vi "Stellarnet_spectrometer_Full_acquire_spectra.vi"() -> ()   [LabVIEW 2014]
uses:
  <vilib>/Utility/file.llb/Write To Spreadsheet File (string).vi
  <vilib>/Utility/file.llb/Write To Spreadsheet File (DBL).vi
panel:
  out "output param":i32
  out "Critical Error":bool
  out "Spectrum":cluster{"Wavelengths":dbl[], "buffer out":sgl[]}(graph)
  in  "Save spectra file path":path=path "C:/Users/User/Desktop/Chamber Data/perovskites/2015-08-04 spectra"
  in  "spectra settings":i32[](array[numeric]) caption="Integration time (ms)\n\nOptical smoothing level\n\nNumber of scans to average\n\nDigitizer clock rate setting" min=0 max=4 step=1
  in  "Aquire spectra":bool
  in  "Seconds between  spectra":dbl caption="Time Target (s)"
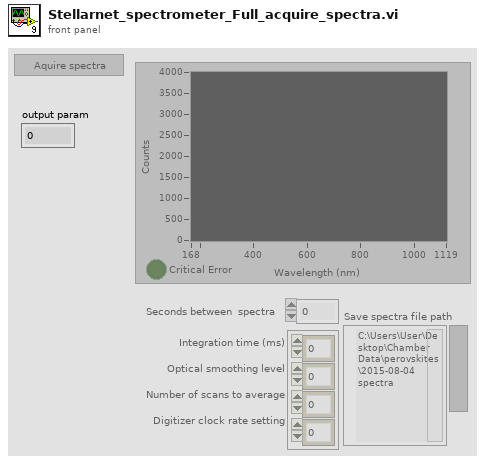
[diagram p1: front panel]
types:
  T1 = enum8{"Enabled", "Disabled", "Disabled and Grayed Out"}
  T2 = cluster{"Coefficients":ext[], "Wavelengths":dbl[]}[]
  T3 = cluster{"Integration Time (ms)":i32, "Number of Scans to Average":i32, "Optical Smoothing Level":i32, "Digitizer Clock Rate Setting":i32, "Temp  Compensation ":bool}[]
  T4 = cluster{"Integration Time (ms)":i32, "Number of Scans to Average":i32, "Optical Smoothing Level":i32, "Digitizer Clock Rate Setting":i32, "Temp  Compensation ":bool}
  T5 = cluster{"Coefficients":ext[], "Wavelengths":dbl[]}
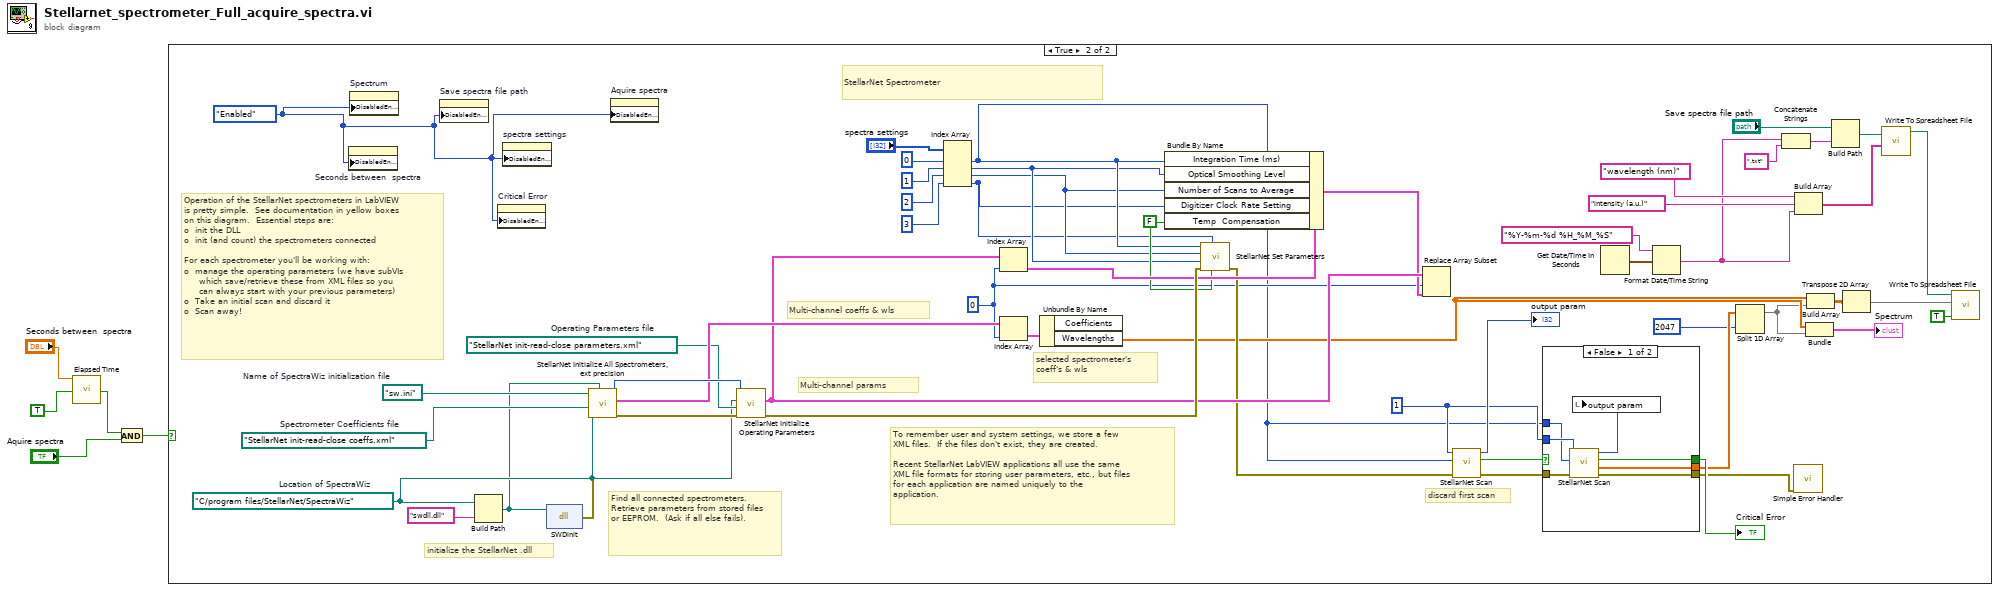
[diagram p0: block diagram]
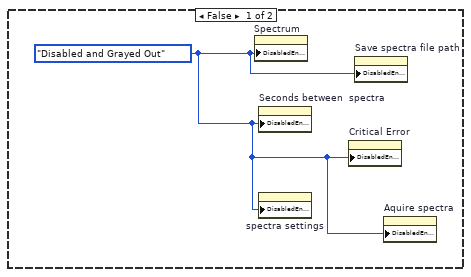
[diagram p2: hidden frame]
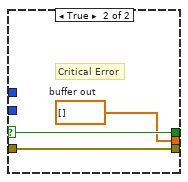
[diagram p3: hidden frame]
diagram:
  n1 = call "Elapsed Time"("Time Target (s)"="Seconds between  spectra", "Auto Reset"=TRUE) -> ("Time has Elapsed"=w3:bool)  [unwired: 10 in, 7 out]
  n2 = And(x=w3, y="Aquire spectra") -> (x .and. y?=w1:bool)
  n3 = case shown="True" w1 {
    frame False {
      w6 = T1."Disabled and Grayed Out" ("Disabled")
      n4 = property on="Spectrum" class="XYGraph (strict)"("DisabledEnum"=w6) -> ()  [unwired: 2 in, 2 out]
      n5 = property on="Seconds between  spectra" class="DigNum (strict)"("DisabledEnum"=w6) -> ()  [unwired: 2 in, 2 out]
      n6 = property on="spectra settings" class="Arr (strict)"("DisabledEnum"=w6) -> ()  [unwired: 2 in, 2 out]
      n7 = property on="Critical Error" class="Bool (strict)"("DisabledEnum"=w6) -> ()  [unwired: 2 in, 2 out]
      n8 = property on="Save spectra file path" class="Path"("DisabledEnum"=w6) -> ()  [unwired: 2 in, 2 out]
      n9 = property on="Aquire spectra" class="Bool (strict)"("DisabledEnum"=w6) -> ()  [unwired: 2 in, 2 out]
    }
    frame True {
      w7 = T1."Enabled" ("Disabled")
      w31 = 0 ("Spectral Channel")
      w33 = 1 ("Spectral Channel")
      w37 = FALSE ("Temp  Compensation")
      w41 = path "C:/program files/StellarNet/SpectraWiz"  # Location of SpectraWiz
      w51 = path "sw.ini"  # Name of SpectraWiz initialization file
      w43 = path "StellarNet init-read-close parameters.xml"  # Operating Parameters file
      w52 = path "StellarNet init-read-close coeffs.xml"  # Spectrometer Coefficients file
      # "StellarNet Spectrometer"
      # "Operation of the StellarNet spectrometers in LabVIEW\nis pretty simple.  See documentation in yellow boxes\non this diagram.  Essential steps are:\no  init the DLL\no  init (and count) the spectrometers connected\n\nFor each spectrometer you'll be working with:\no  manage the operating parameters (we have subVIs\n     which save/retrieve these from XML files so you\n     can always start with your previous parameters)\no  Take an initial scan and discard it\no  Scan away!"
      # "initialize the StellarNet .dll"
      # "To remember user and system settings, we store a few \nXML files.  If the files don't exist, they are created.\n\nRecent StellarNet LabVIEW applications all use the same\nXML file formats for storing user parameters, etc., but files\nfor each application are named uniquely to the \napplication."
      # "Find all connected spectrometers.  Retrieve parameters from stored files or EEPROM.  (Ask if all else fails)."
      # "selected spectrometer's\ncoeff's & wls"
      # "Multi-channel coeffs & wls"
      # "Multi-channel params"
      # "discard first scan"
      n10 = property on="Seconds between  spectra" class="DigNum (strict)"("DisabledEnum"=w7) -> ()  [unwired: 2 in, 2 out]
      n11 = property on="Spectrum" class="XYGraph (strict)"("DisabledEnum"=w7) -> ()  [unwired: 2 in, 2 out]
      n12 = property on="Save spectra file path" class="Path"("DisabledEnum"=w7) -> ()  [unwired: 2 in, 2 out]
      n13 = Build Path(base path=w41, name or relative path="swdll.dll") -> (appended path=w39:path)
      n14 = property on="Critical Error" class="Bool (strict)"("DisabledEnum"=w7) -> ()  [unwired: 2 in, 2 out]
      n15 = property on="spectra settings" class="Arr (strict)"("DisabledEnum"=w7) -> ()  [unwired: 2 in, 2 out]
      n16 = dll-call lib="C:/Program Files/StellarNet/SpectraWiz/swdll.dll" fn="SWDinit" label="init"(path in=w39) -> (error out=w40:errorcluster)  [unwired: 3 in, 1 out]
      n17 = call "StellarNet Initialize All Spectrometers, ext precision.vi"("Path of swdll.dll"=w39, "error in"=w40, "Spectrometer Coefficients file"=w52, "Location of SpectraWiz"=w41, "Name of SpectraWiz initialization file"=w51) -> ("error out"=w50:errorcluster, "Multi Channel Coeffs & WLs"=w48:T2, "Number of Channels"=w49:i32)  [unwired: 2 in, 2 out]
      n18 = property on="Aquire spectra" class="Bool (strict)"("DisabledEnum"=w7) -> ()  [unwired: 2 in, 2 out]
      n19 = call "StellarNet Initialize Operating Parameters.vi"("error in"=w50, "Spectrometer Coefficients file"=w43, "Location of SpectraWiz"=w41, "Number of Channels"=w49) -> ("error out"=w46:errorcluster, "Operating Parameters"=w44:T3)  [unwired: 6 in]
      n20 = Index Array(array="spectra settings", index #1=0 ("index"), index #2=1 ("index"), index #3=2 ("index"), index #4=3 ("index")) -> (element #1=w11:i32, element #2=w10:i32, element #3=w9:i32, element #4=w8:i32)
      n21 = Index Array(array=w44, index=w31) -> (element=w45:T4)
      n22 = Index Array(array=w48, index=w31) -> (element=w47:T5)
      n23 = Unbundle By Name(w47) -> ("Wavelengths"=w35:dbl[])  [unwired: 1 out]
      n24 = Bundle By Name(cluster=w45, "Integration Time (ms)"=w11, "Optical Smoothing Level"=w10, "Number of Scans to Average"=w9, "Digitizer Clock Rate Setting"=w8, "Temp  Compensation"=w37) -> (w38:T4)
      n25 = call "StellarNet Set Parameters.vi"("Temp  Compensation"=w37, "Digitizer Clock Rate Setting"=w8, "error in (no error)"=w46, "Optical Smoothing Level"=w10, "Number of Scans to Average"=w9, "Integration Time (ms)"=w11) -> ("error out"=w36:errorcluster)  [unwired: 5 in]
      n26 = Replace Array Subset(array=w44, new element=w38, index=w31) -> ()  [unwired: 1 out]
      n27 = call "StellarNet Scan.vi"("error in (no error)"=w36, "Integration Time (msec)"=w11, "Spectral Channel"=w33) -> ("error out"=w57:errorcluster, "Critical Error"=w58:bool, "output param"=→"output param":i32)  [unwired: 5 in, 1 out]
      n28 = case shown="False" w58 {
        selector: w58 -> [_ w69]
        tunnel: w33 -> [w66 _]
        tunnel: [w65 w68] -> w42
        tunnel: [w63 w69] -> w55
        tunnel: w57 -> [w62 w67]
        tunnel: [w61 w67] -> w32
        tunnel: w11 -> [w60 _]
        frame False {
          n29 = call "StellarNet Scan.vi"("error in (no error)"=w62, "Integration Time (msec)"=w60, "Spectral Channel"=w66) -> ("error out"=w61:errorcluster, "buffer out"=w65:sgl[], "Critical Error"=w63:bool, "output param"=w64:i32)  [unwired: 5 in]
          n30 = local write "output param"(w64) -> ()
        }
        frame True {
          w68 = sgl[] []  # buffer out
          # "Critical Error"
        }
      }
      "Critical Error" <- w55
      n31 = Get Date/Time In Seconds() -> (seconds since 1Jan1904=w26:timestamp)
      n32 = Format Date/Time String(time format string (%c)="%Y-%m-%d %H_%M_%S", seconds (now)=w26) -> (date/time string=w21:string)  [unwired: 1 in]
      n33 = Split 1D Array(array=w42, index=2047) -> (first subarray=w34:sgl[])  [unwired: 1 out]
      n34 = Concatenate Strings(w21, ".txt") -> (w22:string)
      n35 = call <vilib>:"Simple Error Handler.vi"("error in (no error)"=w32) -> ()  [unwired: 4 in, 5 out]
      n36 = Build Array("wavelength (nm)", "intensity (a.u.)", w21) -> (w17:string[])
      n37 = Bundle("Wavelengths"=w35, w34) -> (→"Spectrum":cluster{"Wavelengths":dbl[], sgl[]})  [unwired: 1 in]
      n38 = Build Array(w35, w34) -> (w20:dbl[][])
      n39 = Build Path(base path="Save spectra file path", name or relative path=w22) -> (appended path=w24:path)
      n40 = Transpose 2D Array(2D array=w20) -> (transposed array=w19:dbl[][])
      n41 = call-poly <vilib>:"Write To Spreadsheet File.vi"("1D data"=w17, "file path (dialog if empty)"=w24) -> ("new file path (Not A Path if cancelled)"=w18:path)  [unwired: 6 in]
      n42 = call-poly <vilib>:"Write To Spreadsheet File.vi"("append to file? (new file:F)"=TRUE, "2D data"=w19, "file path (dialog if empty)"=w18) -> ()  [unwired: 5 in, 1 out]
    }
  }
